vi "Initialize.vi"(8 "error in (no error)":errorcluster, 11 "Sub Panel":refnum<vi>) -> (0 "error out":errorcluster, 3 "Subpanel Manager":refnum<class "SLL Subpanel Manager.lvclass">)   [LabVIEW 2016, in "SLL Subpanel Manager.lvclass"]
uses:
  SLL Subpanel Manager.lvclass
  SLL Subpanel Manager.lvclass/SLL Subpanel Manager.ctl
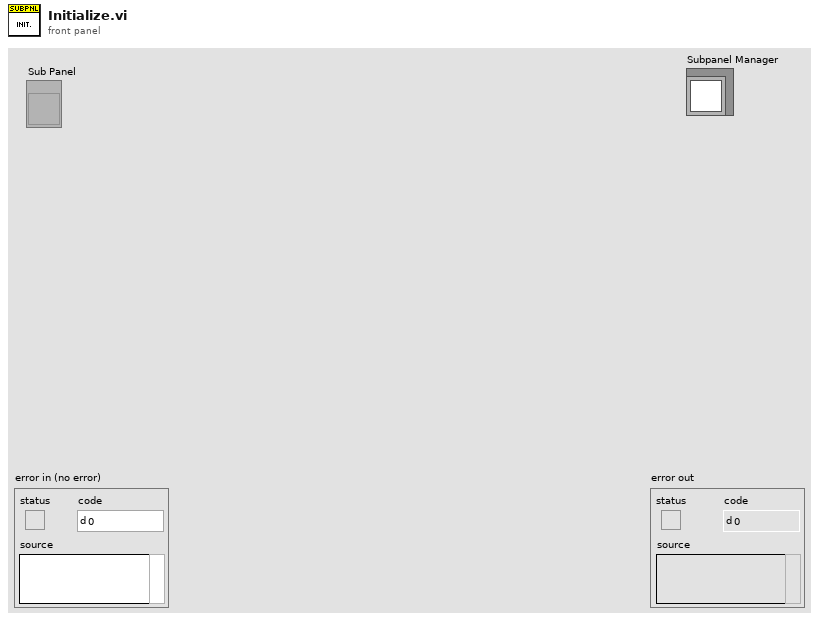
[diagram p1: front panel]
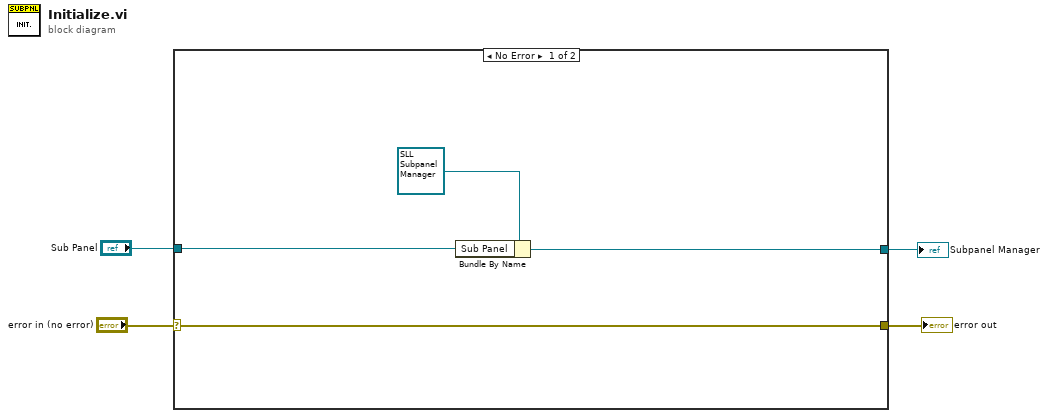
[diagram p0: block diagram]
diagram:
  n1 = case shown="No Error" "error in (no error)" {
    selector: "error in (no error)" -> [w6 w9]
    tunnel: "Sub Panel" -> [w7 _]
    tunnel: [w6 w9] -> w2
    tunnel: [w5 _] -> w1
    frame No Error {
      n2 = Bundle By Name(cluster=refnum<class "SLL Subpanel Manager.lvclass"> refnum ("SLL Subpanel Manager.lvclass"), "Sub Panel"=w7) -> (w5:refnum<class "SLL Subpanel Manager.lvclass">)
    }
    frame Error {
    }
  }
  "error out" <- w2
  "Subpanel Manager" <- w1
